vi "3.1 PositionControlTest (Geared).vi"(6 "Reset":bool, 7 "Position (deg)":dbl(slide) scale=-1000.0..1000.0, 8 "error in (no error)":errorcluster, 11 "Stop Button":bool) -> (0 "error out":errorcluster, 2 "Waveform Chart":T1(graph))   [LabVIEW 2019, in "SJCube.lvlib"]
uses:
  SJCube.lvlib
  <vilib>/Platform/TimedLoop/XDataNode/XDataNode.xnode
  <vilib>/Platform/TimedLoop/XDataNode/nitl_modes.ctl
  <vilib>/Platform/TimedLoop/XDataNode/XDNodeRunTimeDep.lvlib
  <vilib>/Platform/TimedLoop/XDataNode/wakeup.ctl
  <vilib>/Platform/TimedLoop/XDataNode/timing_clust.ctl
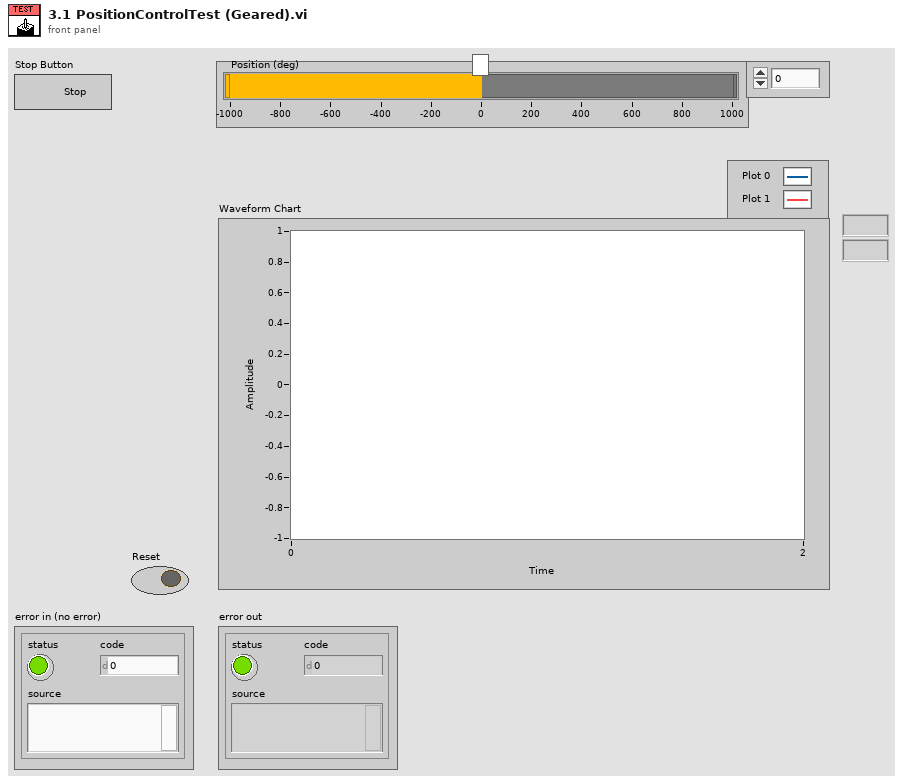
[diagram p1: front panel]
types:
  T1 = cluster{"Position (deg)":dbl, "MotorEncoder (deg)":dbl}
  T2 = typedef "XDNodeRunTimeDep.lvlib/timing_clust.ctl" = cluster{"Expected End [f-1]":u64, "Actual End [f-1]":u64, "Finished Late? [f-1]":bool, "Expected End [i-1]":u64, "Actual End [i-1]":u64, "Finished Late? [i-1]":bool, "Expected Start [i]":u64, "Actual Start [i]":u64, "Expected Start [f]":u64, "Actual Start [f]":u64, "Source Name":string, "Structure Name":string, "Period":i64, "Deadline":i64, "Offset":i64, "Start":i64, "Priority":i32, "Timeout":i32, "Mode":T3, "Wakeup Reason":T4, "Error":errorcluster, "Source Type":string, "Secondary Source Type":string, "Global End Time":u64, "Global Start Time":u64, "Frame Duration":u64, "Iteration Duration":u64, "Assigned CPU":i32, "I/O Scan Engine Mode":u32}
  T3 = typedef "XDNodeRunTimeDep.lvlib/nitl_modes.ctl" = enum32{"No Change", "Process missed periods, maintain original phase", "Discard missed periods, maintain original phase", "Process missed periods, ignore original phase", "Discard missed periods, ignore original phase"}
  T4 = typedef "XDNodeRunTimeDep.lvlib/wakeup.ctl" = enum32{"Normal", "Aborted", "Asynchronous wakeup", "Timing source error", "Timed loop error", "Timeout"}
  T5 = cluster{"proportional gain (Kc)":dbl, "integral time (Ti, min)":dbl, "derivative time (Td, min)":dbl}
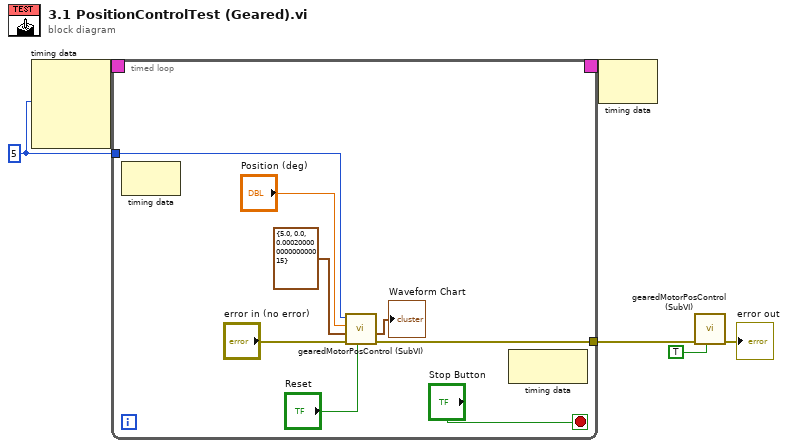
[diagram p0: block diagram]
diagram:
  w1 = i64 5 ("Period")
  n1 = node-c288(w1) -> (w6:T2)  [unwired: 3 in]
  n2 = timed-loop {
    timing: w6 -> [_]
    timing-out: [_] -> w5
    tunnel: [w13] -> w4
    tunnel: w1 -> [w7]
    stop <- "Stop Button" stop-if-true
    n3 = node-c288() -> ()  [unwired: 1 in, 1 out]
    n4 = call "gearedMotorPosControl (SubVI).vi"("Reset"="Reset", "error in (no error)"="error in (no error)", "PID gains"=T5 {"proportional gain (Kc)"=5.0, "integral time (Ti, min)"=0.0, "derivative time (Td, min)"=0.00020000000000000015}, "Position (deg)"="Position (deg)", "dt"=w7) -> ("error out"=w13:errorcluster, "Waveform Chart"=→"Waveform Chart":T1)  [unwired: 4 in, 1 out]
    n5 = node-c288() -> ()  [unwired: 1 in, 1 out]
  }
  n6 = node-c288(w5) -> ()  [unwired: 1 out]
  n7 = call "gearedMotorPosControl (SubVI).vi"("Reset"=TRUE, "error in (no error)"=w4) -> ("error out"=→"error out":errorcluster)  [unwired: 7 in, 2 out]
